vi "test_timeoutErrorValidation.vi"(11 "Test Case In":refnum<class "TaskControllerTests.lvclass">) -> (0 "error out":errorcluster, 3 "Test Case Out":refnum<class "TaskControllerTests.lvclass">)   [LabVIEW 2023, in "TaskControllerTests.lvclass"]
uses:
  TaskControllerTests.lvclass
  TaskMock/TaskMock.lvclass
  C:/projects/TLC_Daemon/source/ITask/ITask.lvclass
  TaskControllerTests.lvclass/TaskControllerTests.ctl
  source/TaskController/TaskController.lvclass
  <vilib>/Astemes/LUnit/Palette/Advanced Assertions/LUnit Advanced Assertions.lvlib
  C:/Program Files (x86)/National Instruments/LabVIEW 2023/vi.lib/Astemes/LUnit/Test Case.lvclass
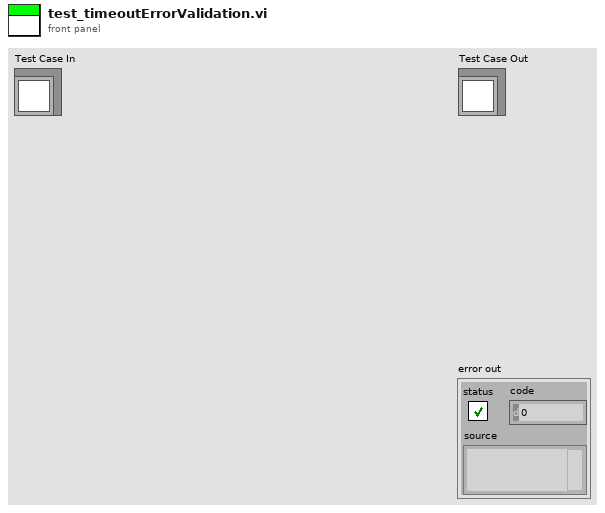
[diagram p1: front panel]
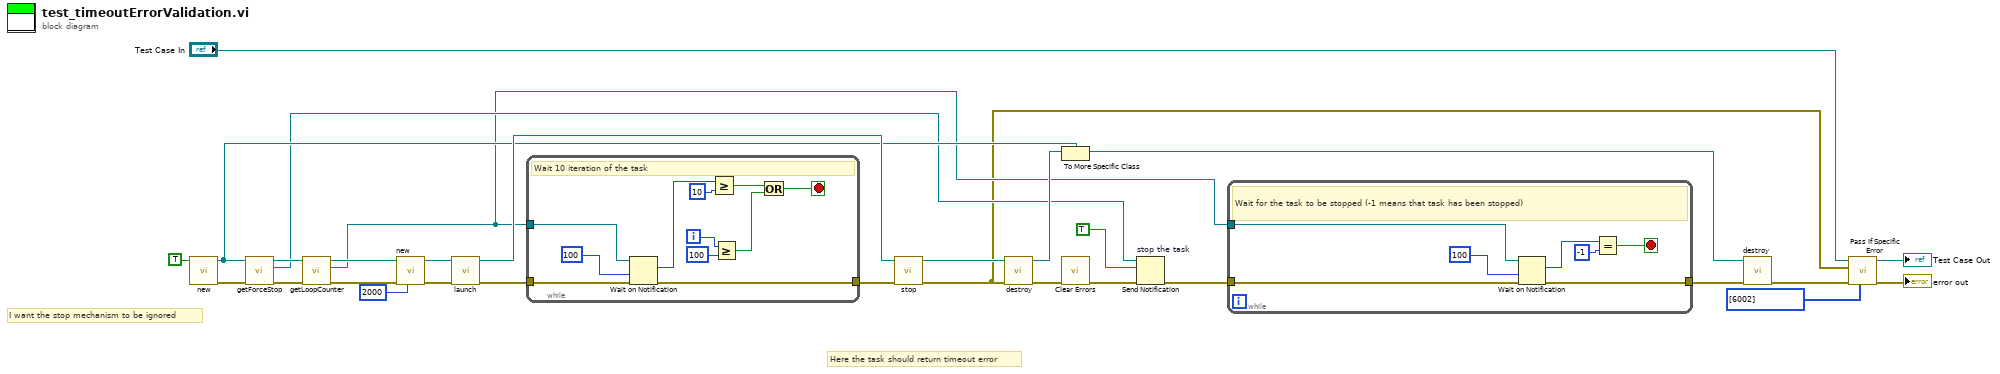
[diagram p0: block diagram]
diagram:
  # "I want the stop mechanism to be ignored"
  # "Here the task should return timeout error"
  n1 = call "new.vi"("ignoreStopMechanism"=TRUE) -> ("error out"=w18:errorcluster, "TaskMock out"=w13:refnum<class "TaskMock.lvclass">)  [unwired: 9 in]
  n2 = call "getForceStop.vi"("error in (no error)"=w18, "TaskMock in"=w13) -> ("error out"=w15:errorcluster, "forceStop"=w8:refnum<notifier>, "TaskMock out"=w14:refnum<class "TaskMock.lvclass">)  [unwired: 7 in]
  n3 = call "getLoopCounter.vi"("error in (no error)"=w15, "TaskMock in"=w14) -> ("error out"=w17:errorcluster, "loopCounter"=w7:refnum<notifier>, "TaskMock out"=w23:refnum<class "TaskMock.lvclass">)  [unwired: 7 in]
  n4 = call "new.vi"("stopTimeout[ms]"=2000, "error in (no error)"=w17, "task"=w23) -> ("error out"=w25:errorcluster, "TaskController out"=w26:refnum<class "TaskController.lvclass">)  [unwired: 7 in]
  n5 = call "launch.vi"("error in (no error)"=w25, "TaskController in"=w26) -> ("error out"=w24:errorcluster, "TaskController out"=w22:refnum<class "TaskController.lvclass">)  [unwired: 8 in]
  n6 = while {
    tunnel: w24 -> [w31]
    tunnel: w7 -> [w40]
    tunnel: [w30] -> w21
    i -> [w36]
    stop <- w33 stop-if-true
    # "Wait 10 iteration of the task"
    n7 = Wait on Notification(notifier=w40, timeout in ms (-1)=100, error in (no error)=w31) -> (notification=w38:i32, error out=w30:errorcluster)  [unwired: 1 in, 2 out]
    n8 = Greater Or Equal?(x=w38, y=10) -> (x >= y?=w34:bool)
    n9 = Greater Or Equal?(x=w36, y=100) -> (x >= y?=w32:bool)
    n10 = Or(x=w34, y=w32) -> (x .or. y?=w33:bool)
  }
  n11 = call "stop.vi"("error in (no error)"=w21, "TaskController in"=w22) -> ("error out"=w2:errorcluster, "TaskController out"=w16:refnum<class "TaskController.lvclass">)  [unwired: 8 in]
  n12 = call "destroy.vi"("error in (no error)"=w2, "TaskController in"=w16) -> ("error out"=w6:errorcluster, "taskResult"=w20:refnum<class "ITask.lvclass">)  [unwired: 8 in]
  n13 = To More Specific Class(target class=w13, reference=w20) -> (specific class reference=w19:refnum<class "TaskMock.lvclass">)  [unwired: 1 in, 1 out]
  n14 = call <vilib>:"Clear Errors.vi"("error in (no error)"=w6) -> ("error out"=w5:errorcluster)  [unwired: 5 in, 1 out]
  n15 = Send Notification "stop the task"(notification=TRUE, notifier=w8, error in (no error)=w5) -> (error out=w9:errorcluster)  [unwired: 1 out]
  n16 = while {
    tunnel: w9 -> [w44]
    tunnel: w7 -> [w47]
    tunnel: [w43] -> w4
    stop <- w41 stop-if-true
    # "Wait for the task to be stopped (-1 means that task has been stopped)"
    n17 = Wait on Notification(notifier=w47, timeout in ms (-1)=100, error in (no error)=w44) -> (notification=w45:i32, error out=w43:errorcluster)  [unwired: 1 in, 2 out]
    n18 = Equal?(x=w45, y=-1) -> (x = y?=w41:bool)
  }
  n19 = call "destroy.vi"("error in (no error)"=w4, "TaskMock in"=w19) -> ("error out"=w3:errorcluster)  [unwired: 9 in]
  n20 = call <vilib>:"Pass If Specific Error.vi"("Error Codes"=i32[] [6002], "error in (no error)"=w3, "Assert error"=w2, "LUnit Test Case In"="Test Case In") -> ("error out"=→"error out":errorcluster, "LUnit Test Case Out"=→"Test Case Out":refnum<class "TaskControllerTests.lvclass">)  [unwired: 6 in]
